vi "defendAreaTacticCheckStateChange.vi"(8 "error in (no error)":errorcluster, 9 "Robot In":refnum<class "Robot.lvclass">, 10 "Game in":refnum<class "Game.lvclass">, 11 "DefendAreaTacticVSS in":refnum<class "DefendAreaTacticVSS.lvclass">) -> (0 "error out":errorcluster, 2 "State":T1(ring), 3 "DefendAreaTacticVSS out":refnum<class "DefendAreaTacticVSS.lvclass">)   [LabVIEW 2020, in "DefendAreaTacticVSS.lvclass"]
uses:
  DefendAreaTacticVSS.lvclass
  Game_class/Game.lvclass
  Robot_class/Robot.lvclass
  C:/Users/lucio/Desktop/Horie/ROBOIME/VSS_AI/Object_class/Object.lvclass
  Game_class/Game.lvclass/Game.ctl
  Object_class/Object.lvclass/Object.ctl
  Team_class/Team.lvclass/Team.ctl
  Object_class/Read x.vi
  Object_class/Read y.vi
  Game_class/Read BallRef.vi
  Game_class/Read EnemyRef.vi
  Game_class/Read KeeperTeam.vi
  Game_class/Read FieldRef.vi
  Team_class/Read RobotRef.vi
  Ally_class/Ally.lvclass
  C:/Users/lucio/Desktop/Horie/ROBOIME/VSS_AI/Team_class/Team.lvclass
  Enemy_class/Enemy.lvclass
  Ball_class/Ball.lvclass
  Field_class/Field.lvclass
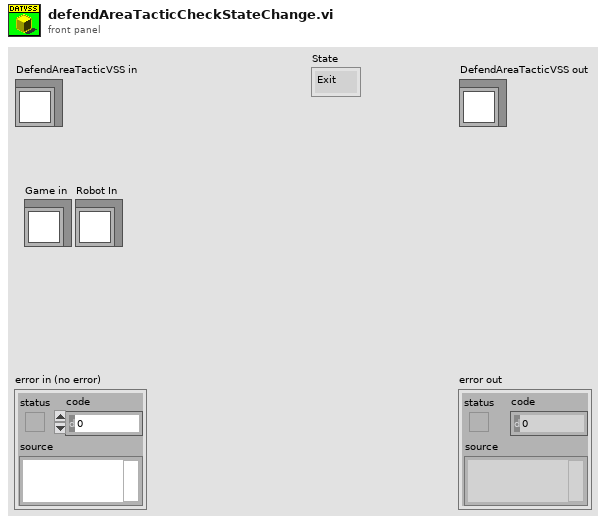
[diagram p1: front panel]
types:
  T1 = enum16{"Exit", "Kick", "DefBallPos", "GoToBall", "Halt"}
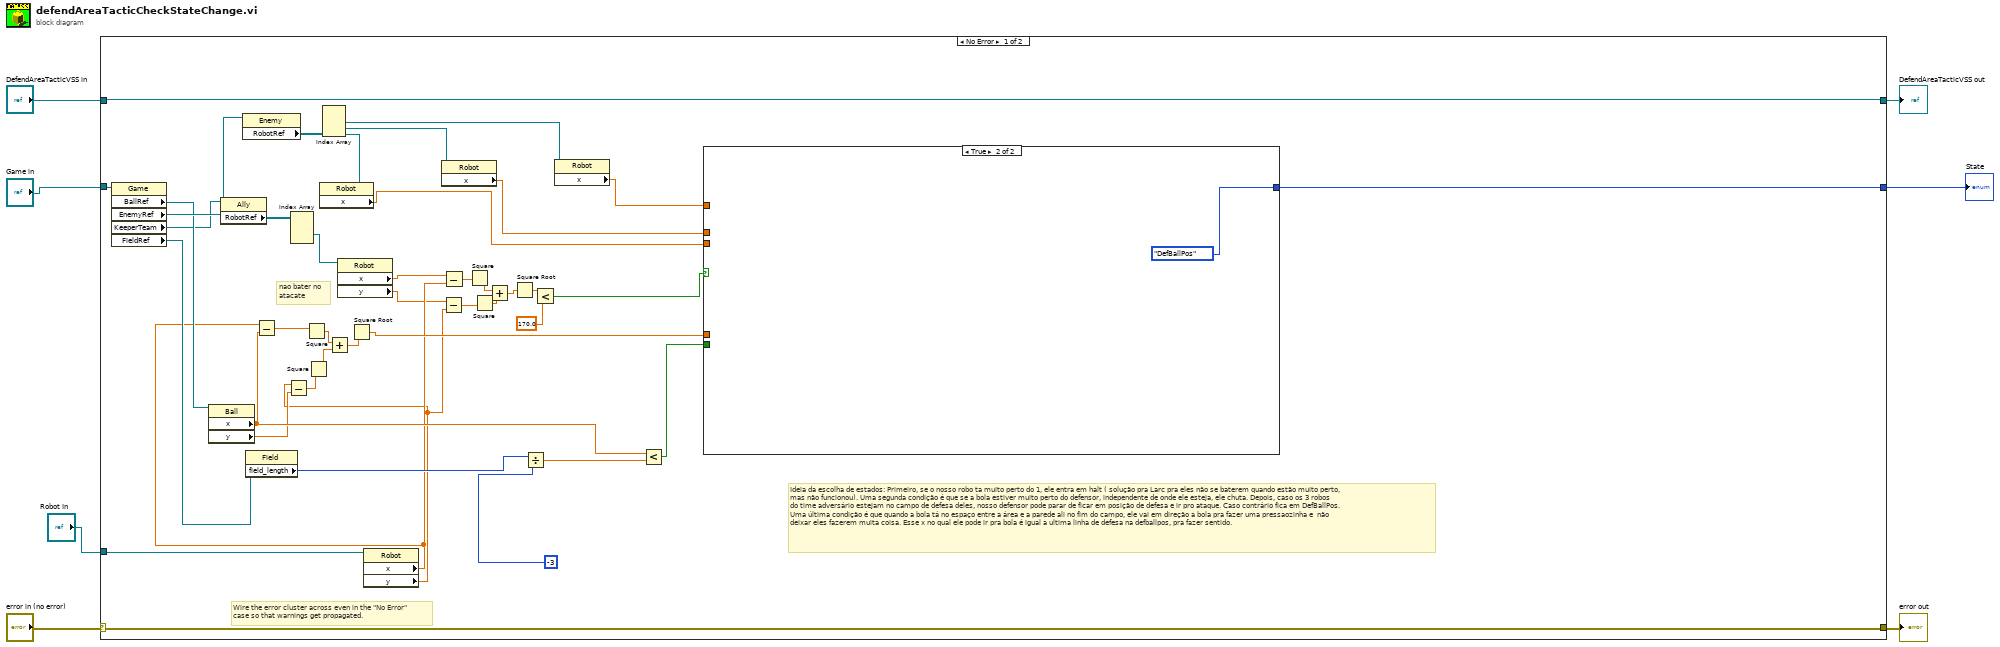
[diagram p0: block diagram]
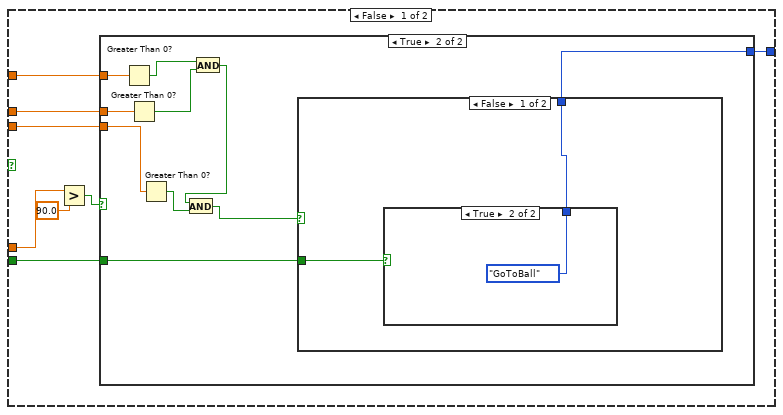
[diagram p2: hidden frame]
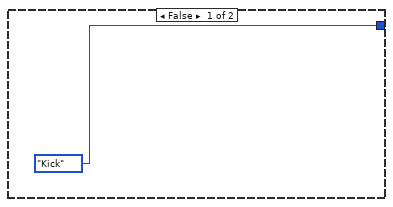
[diagram p3: hidden frame]
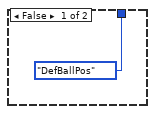
[diagram p4: hidden frame]
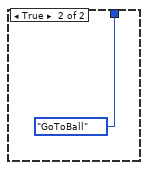
[diagram p5: hidden frame]
diagram:
  n1 = case shown="No Error" "error in (no error)" {
    selector: "error in (no error)" -> [w48 w76]
    tunnel: [w48 w76] -> w6
    tunnel: [w49 w75] -> w4
    tunnel: "DefendAreaTacticVSS in" -> [w49 w75]
    tunnel: "Game in" -> [w47 _]
    tunnel: "Robot In" -> [w36 _]
    tunnel: [w33 _] -> w1
    frame No Error {
      # "Ideia da escolha de estados: Primeiro, se o nosso robo ta muito perto do 1, ele entra em halt ( solução pra Larc pra eles não se baterem quando estão muito perto, \nmas não funcionou). Uma segunda condição é que se a bola estiver muito perto do defensor, independente de onde ele esteja, ele chuta. Depois, caso os 3 robos\ndo time adversário estejam no campo de defesa deles, nosso defensor pode parar de ficar em posição de defesa e ir pro ataque. Caso contrário fica em DefBallPos. \nUma última condição é que quando a bola tá no espaço entre a área e a parede ali no fim do campo, ele vai em direção a bola pra fazer uma pressaozinha e  não \ndeixar eles fazerem muita coisa. Esse x no qual ele pode ir pra bola é igual a ultima linha de defesa na defballpos, pra fazer sentido."
      # "nao bater no\natacate"
      # "Wire the error cluster across even in the \"No Error\"\ncase so that warnings get propagated."
      n2 = property class="Game"(reference=w47) -> ("BallRef"=w43:refnum<class "Ball.lvclass">, "EnemyRef"=w46:refnum<class "Enemy.lvclass">, "KeeperTeam"=w39:refnum<class "Ally.lvclass">, "FieldRef"=w41:refnum<class "Field.lvclass">)  [unwired: 1 in, 2 out]
      n3 = property class="Ball"(reference=w43) -> ("x"=w25:dbl, "y"=w23:dbl)  [unwired: 1 in, 2 out]
      n4 = property class="Ally"(reference=w39) -> ("RobotRef"=w38:refnum<class "Robot.lvclass">[])  [unwired: 1 in, 2 out]
      n5 = property class="Enemy"(reference=w46) -> ("RobotRef"=w45:refnum<class "Robot.lvclass">[])  [unwired: 1 in, 2 out]
      n6 = property class="Field"(reference=w41) -> ("field_length"=w40:i32)  [unwired: 1 in, 2 out]
      n7 = Index Array(array=w38) -> (element #2=w37:refnum<class "Robot.lvclass">)  [unwired: 3 in, 2 out]
      n8 = Index Array(array=w45) -> (element #1=w26:refnum<class "Robot.lvclass">, element #2=w27:refnum<class "Robot.lvclass">, element #3=w44:refnum<class "Robot.lvclass">)  [unwired: 3 in]
      n9 = property class="Robot"(reference=w44) -> ("x"=w30:dbl)  [unwired: 1 in, 2 out]
      n10 = property class="Robot"(reference=w37) -> ("x"=w11:dbl, "y"=w9:dbl)  [unwired: 1 in, 2 out]
      n11 = property class="Robot"(reference=w36) -> ("x"=w10:dbl, "y"=w8:dbl)  [unwired: 1 in, 2 out]
      n12 = Subtract(x=w10, y=w25) -> (x-y=w24:dbl)
      n13 = Subtract(x=w8, y=w23) -> (x-y=w22:dbl)
      n14 = Square(x=w24) -> (x^2=w21:dbl)
      n15 = Square(x=w22) -> (x^2=w20:dbl)
      n16 = Add(x=w21, y=w20) -> (x+y=w19:dbl)
      n17 = Square Root(x=w19) -> (sqrt(x)=w18:dbl)
      n18 = property class="Robot"(reference=w27) -> ("x"=w31:dbl)  [unwired: 1 in, 2 out]
      n19 = Subtract(x=w9, y=w8) -> (x-y=w17:dbl)
      n20 = Subtract(x=w11, y=w10) -> (x-y=w16:dbl)
      n21 = Square(x=w16) -> (x^2=w13:dbl)
      n22 = Square(x=w17) -> (x^2=w12:dbl)
      n23 = Add(x=w13, y=w12) -> (x+y=w14:dbl)
      n24 = Square Root(x=w14) -> (sqrt(x)=w15:dbl)
      n25 = Divide(x=w40, y=-3) -> (x/y=w29:dbl)
      n26 = Less?(x=w15, y=170.0) -> (x < y?=w34:bool)
      n27 = property class="Robot"(reference=w26) -> ("x"=w32:dbl)  [unwired: 1 in, 2 out]
      n28 = Less?(x=w25, y=w29) -> (x < y?=w28:bool)
      n29 = case shown="True" w34 {
        tunnel: [w54 T1."DefBallPos" ("State")] -> w33
        tunnel: w32 -> [w57 _]
        tunnel: w31 -> [w56 _]
        tunnel: w30 -> [w55 _]
        tunnel: w28 -> [w53 _]
        tunnel: w18 -> [w50 _]
        frame False {
          n30 = Greater?(x=w50, y=90.0) -> (0:w52:bool)
          n31 = case shown="True" w52 {
            tunnel: w57 -> [_ w68]
            tunnel: w56 -> [_ w66]
            tunnel: w55 -> [_ w64]
            tunnel: [T1."Kick" ("State") w60] -> w54
            tunnel: w53 -> [_ w59]
            frame False {
            }
            frame True {
              n32 = Greater Than 0?(x=w68) -> (x > 0?=w67:bool)
              n33 = Greater Than 0?(x=w66) -> (x > 0?=w65:bool)
              n34 = Greater Than 0?(x=w64) -> (x > 0?=w62:bool)
              n35 = And(x=w67, y=w65) -> (x .and. y?=w63:bool)
              n36 = And(x=w63, y=w62) -> (x .and. y?=w61:bool)
              n37 = case shown="False" w61 {
                tunnel: [w69 T1."GoToBall" ("State")] -> w60
                tunnel: w59 -> [w70 _]
                frame False {
                  n38 = case shown="True" w70 {
                    tunnel: [T1."DefBallPos" ("State") T1."GoToBall" ("State")] -> w69
                    frame False {
                    }
                    frame True {
                    }
                  }
                }
                frame True {
                }
              }
            }
          }
        }
        frame True {
        }
      }
    }
    frame Error {
    }
  }
  "error out" <- w6
  "DefendAreaTacticVSS out" <- w4
  "State" <- w1
